vi "Get Timestamp.vi"(0 "reference in":refnum<class "Grapher.lvclass">, 5 "Error In":errorcluster) -> (14 "reference out":refnum<class "Grapher.lvclass">, 16 "timestamp (seconds)":dbl, 19 "Error Out":errorcluster)   [LabVIEW 2023, in "Grapher.lvclass"]
uses:
  Grapher.lvclass
  Grapher.lvclass/Grapher.ctl
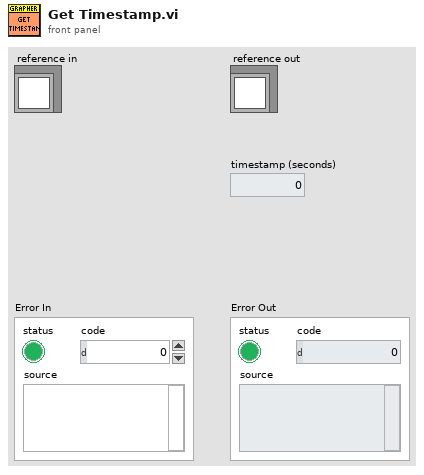
[diagram p1: front panel]
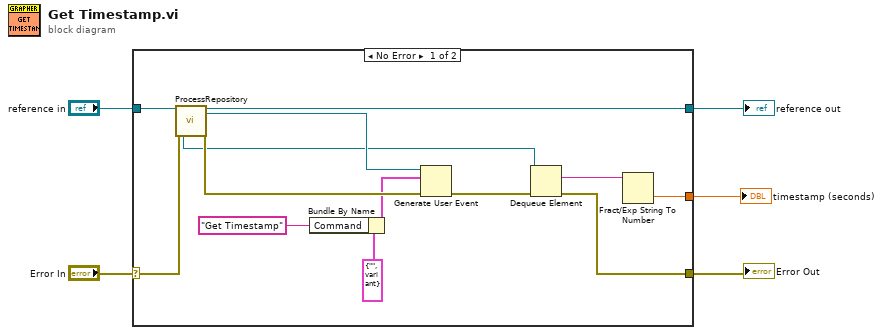
[diagram p0: block diagram]
diagram:
  n1 = case shown="No Error" "Error In" {
    selector: "Error In" -> [w18 w20]
    tunnel: [w12 w20] -> w4
    tunnel: [w16 w19] -> w2
    tunnel: "reference in" -> [w17 w19]
    tunnel: [w6 _] -> w1
    frame No Error {
      n2 = call "ProcessRepository.vi"("reference in"=w17, "Error In"=w18) -> ("QueueFromProcess"=w9:refnum<queue>, "reference out"=w16:refnum<class "Grapher.lvclass">, "EventsToProcess"=w15:refnum<user-event>, "Error Out"=w13:errorcluster)  [unwired: 10 in, 4 out]
      n3 = Bundle By Name(cluster=cluster{"Command":string, "Data":variant} {"Command"="", "Data"=variant} ("MessageToProcess"), "Command"="Get Timestamp") -> (w10:cluster{"Command":string, "Data":variant})
      n4 = Generate User Event(user event=w15, event data cluster=w10, error in=w13) -> (error out=w14:errorcluster)  [unwired: 1 in, 1 out]
      n5 = Dequeue Element(queue=w9, error in (no error)=w14) -> (element=w7:string, error out=w12:errorcluster)  [unwired: 1 in, 2 out]
      n6 = Fract/Exp String To Number(string=w7) -> (number=w6:dbl)  [unwired: 3 in, 1 out]
    }
    frame Error {
    }
  }
  "Error Out" <- w4
  "reference out" <- w2
  "timestamp (seconds)" <- w1
